vi "QDMH Get or Obtain Queue.vi"(8 "error in (no error)":errorcluster, 10 "Queue Name":string, 11 "VI Refnum":refnum<vi>) -> (0 "error out":errorcluster, 2 "Created New?":bool, 3 "queue out":refnum<queue>)   [LabVIEW 2009]
doc: "This VI will parse a command from the data variant and display both.\n\nAAL 9/09"
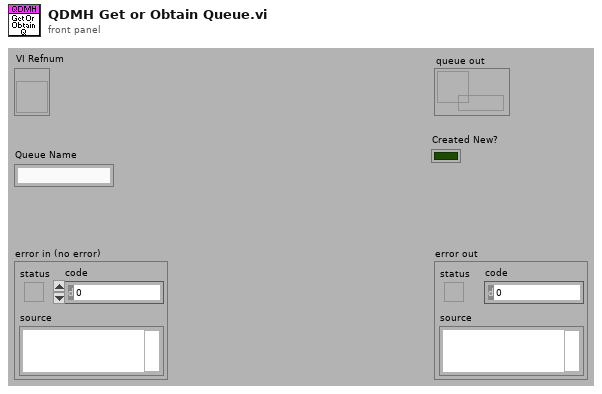
[diagram p1: front panel]
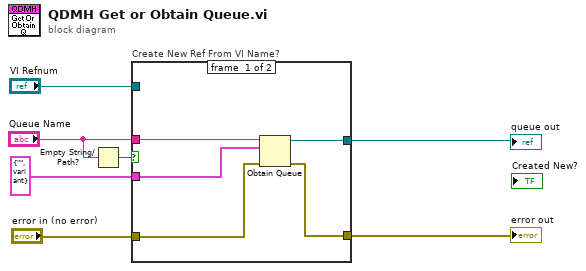
[diagram p0: block diagram]
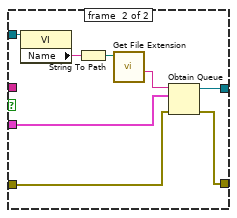
[diagram p2: hidden frame]
diagram:
  n1 = Empty String/Path?(string/path="Queue Name") -> (empty?=w4:bool)
  n2 = case "Create New Ref From VI Name?" shown="True" w4 {
    tunnel: "error in (no error)" -> [w12 w20]
    tunnel: [w11 w19] -> w6
    tunnel: [w10 w18] -> w5
    tunnel: "Queue Name" -> [w9 _]
    tunnel: cluster{"State":string, "Variant Data":variant} {"State"="", "Variant Data"=variant} ("QDSM Element") -> [w8 w17]
    tunnel: "VI Refnum" -> [_ w16]
    frame #0 {
      n3 = Obtain Queue(name (unnamed)=w9, element data type=w8, error in (no error)=w12) -> (queue out=w10:refnum<queue>, error out=w11:errorcluster)  [unwired: 2 in, 1 out]
    }
    frame #1 {
      n4 = property class="VI"(reference=w16) -> ("Name"=w14:string)  [unwired: 1 in, 2 out]
      n5 = String To Path(string=w14) -> (path=w13:path)
      n6 = call <vilib>:"Get File Extension.vi"("file"=w13) -> ("filename without extension"=w15:string)  [unwired: 1 in, 9 out]
      n7 = Obtain Queue(name (unnamed)=w15, element data type=w17, error in (no error)=w20) -> (queue out=w18:refnum<queue>, error out=w19:errorcluster)  [unwired: 2 in, 1 out]
    }
  }
  "error out" <- w6
  "queue out" <- w5
